vi "read shared memory.vi"(6 "channel classification":T1, 8 "error in":errorcluster, 10 "data table":T2, 11 "Shared Memory runtime":refnum<class "Shared Memory runtime.lvclass">) -> (0 "error out":errorcluster, 2 "data table out":T2, 3 "Shared Memory runtime out":refnum<class "Shared Memory runtime.lvclass">)   [LabVIEW 2014, in "Shared Memory runtime.lvclass"]
uses:
  Shared Memory runtime.lvclass
  <vilib>/NI/Tag Bus/table/data table.ctl
  <vilib>/NI/Tag Bus Module Framework/channel/channel classification.ctl
  Shared Memory runtime.lvclass/Shared Memory runtime.ctl
  <vilib>/NI/Tag Bus/table/data polymorphs/write many/write Doubles.vi
  <vilib>/NI/Tag Bus/table/data polymorphs/write many/write Singles.vi
  <vilib>/NI/Tag Bus/table/data polymorphs/write many/write I64s.vi
  <vilib>/NI/Tag Bus/table/data polymorphs/write many/write I32s.vi
  <vilib>/NI/Tag Bus/table/data polymorphs/write many/write I16s.vi
  <vilib>/NI/Tag Bus/table/data polymorphs/write many/write I8s.vi
  <vilib>/NI/Tag Bus/table/data polymorphs/write many/write U64s.vi
  <vilib>/NI/Tag Bus/table/data polymorphs/write many/write U32s.vi
  <vilib>/NI/Tag Bus/table/data polymorphs/write many/write U16s.vi
  <vilib>/NI/Tag Bus/table/data polymorphs/write many/write U8s.vi
  <vilib>/NI/Tag Bus/table/data polymorphs/write many/write Booleans.vi
  <vilib>/NI/Tag Bus/table/data polymorphs/write sequential/write sequential Doubles.vi
  <vilib>/NI/Tag Bus/table/data polymorphs/write sequential/write sequential Singles.vi
  <vilib>/NI/Tag Bus/table/data polymorphs/write sequential/write sequential I64s.vi
  <vilib>/NI/Tag Bus/table/data polymorphs/write sequential/write sequential I32s.vi
  <vilib>/NI/Tag Bus/table/data polymorphs/write sequential/write sequential I16s.vi
  <vilib>/NI/Tag Bus/table/data polymorphs/write sequential/write sequential I8s.vi
  <vilib>/NI/Tag Bus/table/data polymorphs/write sequential/write sequential U64s.vi
  <vilib>/NI/Tag Bus/table/data polymorphs/write sequential/write sequential U32s.vi
  <vilib>/NI/Tag Bus/table/data polymorphs/write sequential/write sequential U16s.vi
  <vilib>/NI/Tag Bus/table/data polymorphs/write sequential/write sequential U8s.vi
  <vilib>/NI/Tag Bus/table/data polymorphs/write sequential/write sequential Booleans.vi
  Read input data.vi
  Read processing parameters.vi
  Read processing results.vi
  Read output data.vi
  <vilib>/NI/NI Linux RT IPC/Shared Memory/Classes/Shared Memory/Shared Memory.lvclass
  <vilib>/NI/Tag Bus/table/data table.lvlib
  <vilib>/NI/NI Linux RT IPC/Shared Memory/Shared Memory.lvlib
  <vilib>/NI/Tag Bus Module Framework/channel/TBM channel.lvclass
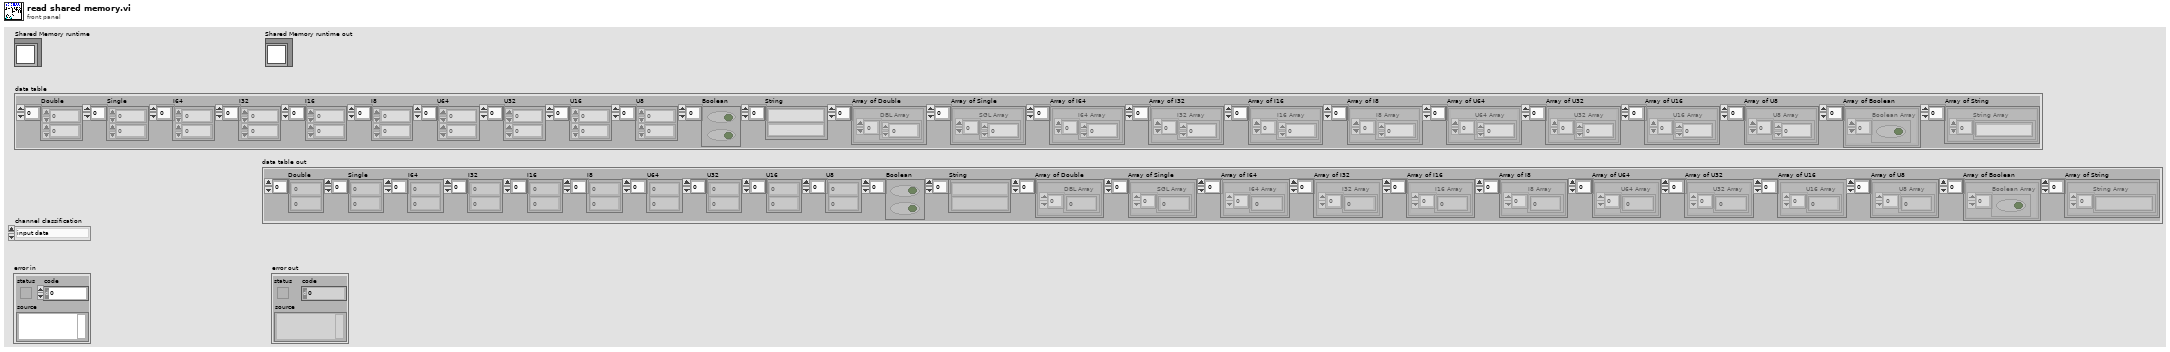
[diagram p1: front panel]
types:
  T1 = typedef "TBM channel.lvclass/channel classification.ctl" = enum16{"input data", "output data", "processing parameter", "processing result"}
  T2 = typedef "tag bus.lvlib/data table.lvlib/data table.ctl" = cluster{"Double":dbl[], "Single":sgl[], "I64":i64[], "I32":i32[], "I16":i16[], "I8":i8[], "U64":u64[], "U32":u32[], "U16":u16[], "U8":u8[], "Boolean":bool[], "String":string[], "Array of Double":cluster{"DBL Array":dbl[]}[], "Array of Single":cluster{"SGL Array":sgl[]}[], "Array of I64":cluster{"I64 Array":i64[]}[], "Array of I32":cluster{"I32 Array":i32[]}[], "Array of I16":cluster{"I16 Array":i16[]}[], "Array of I8":cluster{"I8 Array":i8[]}[], "Array of U64":cluster{"U64 Array":u64[]}[], "Array of U32":cluster{"U32 Array":u32[]}[], "Array of U16":cluster{"U16 Array":u16[]}[], "Array of U8":cluster{"U8 Array":u8[]}[], "Array of Boolean":cluster{"Boolean Array":bool[]}[], "Array of String":cluster{"String Array":string[]}[]}
  T3 = typedef "Shared Memory runtime.lvclass/channel runtime.ctl" = cluster{"channel classification":T1, "data type":T4, "pointer to shared memory":u64, "number of elements":u64, "data dictionary index":cluster{i32[]}, "shared memory":T5, "first tag index":i32, "sequential tags?":bool}
  T4 = typedef "tag bus.lvlib/tag descriptor.lvclass/Data Type.ctl" = enum16{"Double", "Single", "I64", "I32", "I16", "I8", "U64", "U32", "U16", "U8", "Boolean", "String", "Array of Double", "Array of Single", "Array of I64", "Array of I32", "Array of I16", "Array of I8", "Array of U64", "Array of U32", "Array of U16", "Array of U8", "Array of Boolean", "Array of String"}
  T5 = typedef "Linux RT IPC.lvlib/Shared Memory.lvlib/reference.ctl" = refnum<data-value>
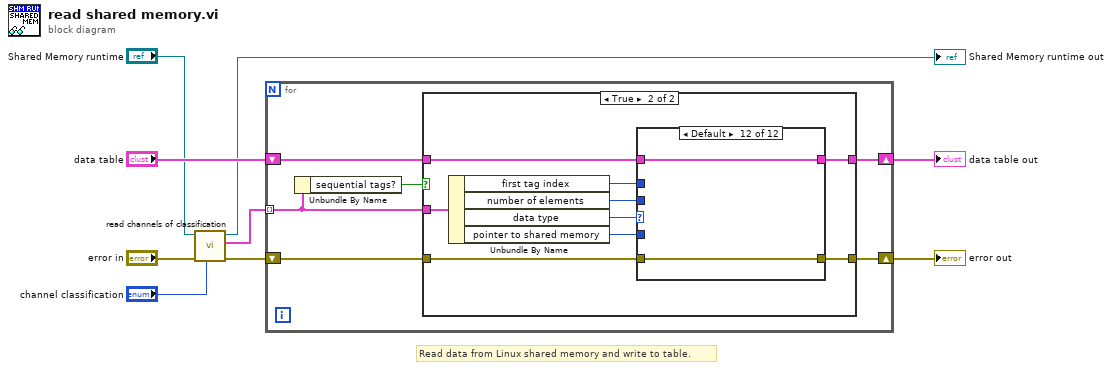
[diagram p0: block diagram]
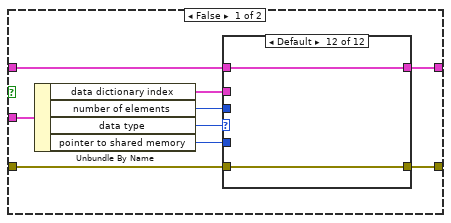
[diagram p2: hidden frame]
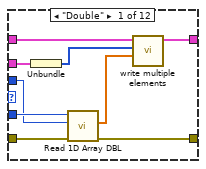
[diagram p3: hidden frame]
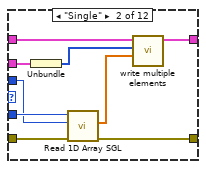
[diagram p4: hidden frame]
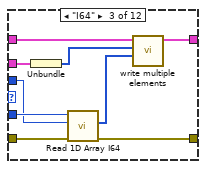
[diagram p5: hidden frame]
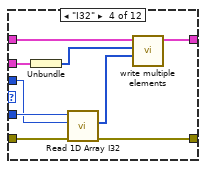
[diagram p6: hidden frame]
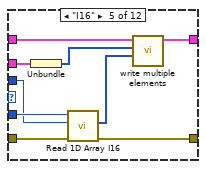
[diagram p7: hidden frame]
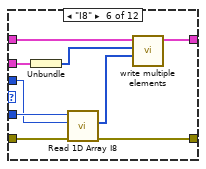
[diagram p8: hidden frame]
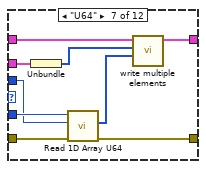
[diagram p9: hidden frame]
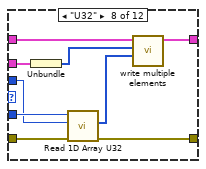
[diagram p10: hidden frame]
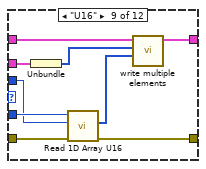
[diagram p11: hidden frame]
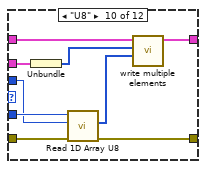
[diagram p12: hidden frame]
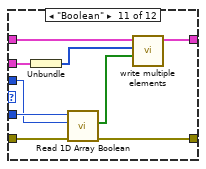
[diagram p13: hidden frame]
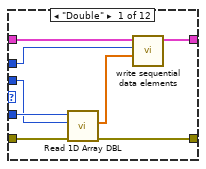
[diagram p14: hidden frame]
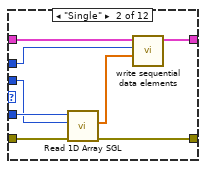
[diagram p15: hidden frame]
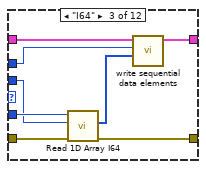
[diagram p16: hidden frame]
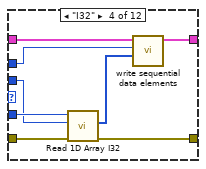
[diagram p17: hidden frame]
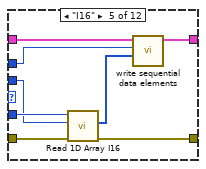
[diagram p18: hidden frame]
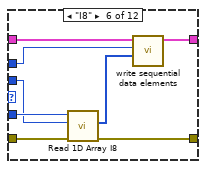
[diagram p19: hidden frame]
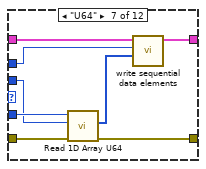
[diagram p20: hidden frame]
diagram:
  # "Read data from Linux shared memory and write to table."
  n1 = call "read channels of classification.vi"("channel classification"="channel classification", "error in"="error in", "Shared Memory runtime in"="Shared Memory runtime") -> ("error out"=w9:errorcluster, "channels"=w8:T3[], "Shared Memory runtime out"=→"Shared Memory runtime out":refnum<class "Shared Memory runtime.lvclass">)  [unwired: 6 in]
  n2 = for {
    tunnel: w8 -> [w11] mode=indexing
    shift-right: [w12] -> w5
    shift-left: w9 -> [w13]
    shift-right: [w15] -> w4
    shift-left: "data table" -> [w14]
    # "Write data from data table to Linux shared memory."
    n3 = Unbundle By Name(w11) -> ("sequential tags?"=w10:bool)
    n4 = case shown="True" w10 {
      tunnel: [w20 w130] -> w15
      tunnel: w14 -> [w21 w131]
      tunnel: w13 -> [w23 w133]
      tunnel: [w22 w132] -> w12
      tunnel: w11 -> [w24 w134]
      frame False {
        n5 = Unbundle By Name(w24) -> ("data dictionary index"=w17:cluster{i32[]}, "number of elements"=w16:u64, "data type"=w18:T4, "pointer to shared memory"=w19:u64)
        n6 = case shown="Default" w18 {
          tunnel: w21 -> [w33 w42 w51 w60 w69 w78 w87 w96 w105 w114 w123 w125]
          tunnel: [w32 w41 w50 w59 w68 w77 w86 w95 w104 w113 w122 w125] -> w20
          tunnel: w23 -> [w30 w39 w48 w57 w66 w75 w84 w93 w102 w111 w121 w124]
          tunnel: [w29 w38 w47 w56 w65 w74 w83 w92 w101 w110 w120 w124] -> w22
          tunnel: w19 -> [w28 w35 w44 w53 w63 w71 w80 w89 w98 w107 w118 _]
          tunnel: w17 -> [w26 w37 w46 w55 w64 w73 w82 w90 w100 w109 w116 _]
          tunnel: w16 -> [w27 w34 w43 w52 w62 w70 w79 w88 w97 w106 w117 _]
          frame "Double" {
            n7 = Unbundle(w26) -> (w25:i32[])
            n8 = call <vilib>:"Read 1D Array DBL.vi"("error in (no error)"=w30, "number of elements"=w27, "pointer in"=w28) -> ("error out"=w29:errorcluster, "value"=w31:dbl[])  [unwired: 6 in, 1 out]
            n9 = call-poly <vilib>:"write multiple elements.vi"("values"=w31, "indices"=w25, "data table in"=w33) -> ("data table out"=w32:T2)  [unwired: 8 in]
          }
          frame "Single" {
            n10 = Unbundle(w37) -> (w36:i32[])
            n11 = call <vilib>:"Read 1D Array SGL.vi"("error in (no error)"=w39, "number of elements"=w34, "pointer in"=w35) -> ("error out"=w38:errorcluster, "value"=w40:sgl[])  [unwired: 6 in, 1 out]
            n12 = call-poly <vilib>:"write multiple elements.vi"("values"=w40, "indices"=w36, "data table in"=w42) -> ("data table out"=w41:T2)  [unwired: 8 in]
          }
          frame "I64" {
            n13 = Unbundle(w46) -> (w45:i32[])
            n14 = call <vilib>:"Read 1D Array I64.vi"("error in (no error)"=w48, "number of elements"=w43, "pointer in"=w44) -> ("error out"=w47:errorcluster, "value"=w49:i64[])  [unwired: 6 in, 1 out]
            n15 = call-poly <vilib>:"write multiple elements.vi"("values"=w49, "indices"=w45, "data table in"=w51) -> ("data table out"=w50:T2)  [unwired: 8 in]
          }
          frame "I32" {
            n16 = Unbundle(w55) -> (w54:i32[])
            n17 = call <vilib>:"Read 1D Array I32.vi"("error in (no error)"=w57, "number of elements"=w52, "pointer in"=w53) -> ("error out"=w56:errorcluster, "value"=w58:i32[])  [unwired: 6 in, 1 out]
            n18 = call-poly <vilib>:"write multiple elements.vi"("values"=w58, "indices"=w54, "data table in"=w60) -> ("data table out"=w59:T2)  [unwired: 8 in]
          }
          frame "I16" {
            n19 = Unbundle(w64) -> (w61:i32[])
            n20 = call <vilib>:"Read 1D Array I16.vi"("error in (no error)"=w66, "number of elements"=w62, "pointer in"=w63) -> ("error out"=w65:errorcluster, "value"=w67:i16[])  [unwired: 6 in, 1 out]
            n21 = call-poly <vilib>:"write multiple elements.vi"("values"=w67, "indices"=w61, "data table in"=w69) -> ("data table out"=w68:T2)  [unwired: 8 in]
          }
          frame "I8" {
            n22 = Unbundle(w73) -> (w72:i32[])
            n23 = call <vilib>:"Read 1D Array I8.vi"("error in (no error)"=w75, "number of elements"=w70, "pointer in"=w71) -> ("error out"=w74:errorcluster, "value"=w76:i8[])  [unwired: 6 in, 1 out]
            n24 = call-poly <vilib>:"write multiple elements.vi"("values"=w76, "indices"=w72, "data table in"=w78) -> ("data table out"=w77:T2)  [unwired: 8 in]
          }
          frame "U64" {
            n25 = Unbundle(w82) -> (w81:i32[])
            n26 = call <vilib>:"Read 1D Array U64.vi"("error in (no error)"=w84, "number of elements"=w79, "pointer in"=w80) -> ("error out"=w83:errorcluster, "value"=w85:u64[])  [unwired: 6 in, 1 out]
            n27 = call-poly <vilib>:"write multiple elements.vi"("values"=w85, "indices"=w81, "data table in"=w87) -> ("data table out"=w86:T2)  [unwired: 8 in]
          }
          frame "U32" {
            n28 = Unbundle(w90) -> (w91:i32[])
            n29 = call <vilib>:"Read 1D Array U32.vi"("error in (no error)"=w93, "number of elements"=w88, "pointer in"=w89) -> ("error out"=w92:errorcluster, "value"=w94:u32[])  [unwired: 6 in, 1 out]
            n30 = call-poly <vilib>:"write multiple elements.vi"("values"=w94, "indices"=w91, "data table in"=w96) -> ("data table out"=w95:T2)  [unwired: 8 in]
          }
          frame "U16" {
            n31 = Unbundle(w100) -> (w99:i32[])
            n32 = call <vilib>:"Read 1D Array U16.vi"("error in (no error)"=w102, "number of elements"=w97, "pointer in"=w98) -> ("error out"=w101:errorcluster, "value"=w103:u16[])  [unwired: 6 in, 1 out]
            n33 = call-poly <vilib>:"write multiple elements.vi"("values"=w103, "indices"=w99, "data table in"=w105) -> ("data table out"=w104:T2)  [unwired: 8 in]
          }
          frame "U8" {
            n34 = Unbundle(w109) -> (w108:i32[])
            n35 = call <vilib>:"Read 1D Array U8.vi"("error in (no error)"=w111, "number of elements"=w106, "pointer in"=w107) -> ("error out"=w110:errorcluster, "value"=w112:u8[])  [unwired: 6 in, 1 out]
            n36 = call-poly <vilib>:"write multiple elements.vi"("values"=w112, "indices"=w108, "data table in"=w114) -> ("data table out"=w113:T2)  [unwired: 8 in]
          }
          frame "Boolean" {
            n37 = Unbundle(w116) -> (w115:i32[])
            n38 = call <vilib>:"Read 1D Array Boolean.vi"("error in (no error)"=w121, "number of elements"=w117, "pointer in"=w118) -> ("error out"=w120:errorcluster, "value"=w119:bool[])  [unwired: 6 in, 1 out]
            n39 = call-poly <vilib>:"write multiple elements.vi"("values"=w119, "indices"=w115, "data table in"=w123) -> ("data table out"=w122:T2)  [unwired: 8 in]
          }
          frame Default {
          }
        }
      }
      frame True {
        n40 = Unbundle By Name(w134) -> ("first tag index"=w127:i32, "number of elements"=w126:u64, "data type"=w128:T4, "pointer to shared memory"=w129:u64)
        n41 = case shown="Default" w128 {
          tunnel: w131 -> [w142 w150 w158 w166 w174 w182 w190 w198 w206 w214 w222 w224]
          tunnel: [w141 w149 w157 w165 w173 w181 w189 w197 w205 w213 w221 w224] -> w130
          tunnel: w133 -> [w139 w147 w155 w163 w171 w179 w187 w195 w203 w211 w220 w223]
          tunnel: [w138 w146 w154 w162 w170 w178 w186 w194 w202 w210 w219 w223] -> w132
          tunnel: w129 -> [w137 w145 w153 w161 w169 w177 w185 w193 w201 w209 w218 _]
          tunnel: w127 -> [w135 w143 w151 w159 w167 w175 w183 w191 w199 w207 w215 _]
          tunnel: w126 -> [w136 w144 w152 w160 w168 w176 w184 w192 w200 w208 w217 _]
          frame "Double" {
            n42 = call <vilib>:"Read 1D Array DBL.vi"("error in (no error)"=w139, "number of elements"=w136, "pointer in"=w137) -> ("error out"=w138:errorcluster, "value"=w140:dbl[])  [unwired: 6 in, 1 out]
            n43 = call-poly <vilib>:"write sequential data elements.vi"("values"=w140, "index"=w135, "data table in"=w142) -> ("data table out"=w141:T2)  [unwired: 8 in]
          }
          frame "Single" {
            n44 = call <vilib>:"Read 1D Array SGL.vi"("error in (no error)"=w147, "number of elements"=w144, "pointer in"=w145) -> ("error out"=w146:errorcluster, "value"=w148:sgl[])  [unwired: 6 in, 1 out]
            n45 = call-poly <vilib>:"write sequential data elements.vi"("values"=w148, "index"=w143, "data table in"=w150) -> ("data table out"=w149:T2)  [unwired: 8 in]
          }
          frame "I64" {
            n46 = call <vilib>:"Read 1D Array I64.vi"("error in (no error)"=w155, "number of elements"=w152, "pointer in"=w153) -> ("error out"=w154:errorcluster, "value"=w156:i64[])  [unwired: 6 in, 1 out]
            n47 = call-poly <vilib>:"write sequential data elements.vi"("values"=w156, "index"=w151, "data table in"=w158) -> ("data table out"=w157:T2)  [unwired: 8 in]
          }
          frame "I32" {
            n48 = call <vilib>:"Read 1D Array I32.vi"("error in (no error)"=w163, "number of elements"=w160, "pointer in"=w161) -> ("error out"=w162:errorcluster, "value"=w164:i32[])  [unwired: 6 in, 1 out]
            n49 = call-poly <vilib>:"write sequential data elements.vi"("values"=w164, "index"=w159, "data table in"=w166) -> ("data table out"=w165:T2)  [unwired: 8 in]
          }
          frame "I16" {
            n50 = call <vilib>:"Read 1D Array I16.vi"("error in (no error)"=w171, "number of elements"=w168, "pointer in"=w169) -> ("error out"=w170:errorcluster, "value"=w172:i16[])  [unwired: 6 in, 1 out]
            n51 = call-poly <vilib>:"write sequential data elements.vi"("values"=w172, "index"=w167, "data table in"=w174) -> ("data table out"=w173:T2)  [unwired: 8 in]
          }
          frame "I8" {
            n52 = call <vilib>:"Read 1D Array I8.vi"("error in (no error)"=w179, "number of elements"=w176, "pointer in"=w177) -> ("error out"=w178:errorcluster, "value"=w180:i8[])  [unwired: 6 in, 1 out]
            n53 = call-poly <vilib>:"write sequential data elements.vi"("values"=w180, "index"=w175, "data table in"=w182) -> ("data table out"=w181:T2)  [unwired: 8 in]
          }
          frame "U64" {
            n54 = call <vilib>:"Read 1D Array U64.vi"("error in (no error)"=w187, "number of elements"=w184, "pointer in"=w185) -> ("error out"=w186:errorcluster, "value"=w188:u64[])  [unwired: 6 in, 1 out]
            n55 = call-poly <vilib>:"write sequential data elements.vi"("values"=w188, "index"=w183, "data table in"=w190) -> ("data table out"=w189:T2)  [unwired: 8 in]
          }
          frame "U32" {
            n56 = call <vilib>:"Read 1D Array U32.vi"("error in (no error)"=w195, "number of elements"=w192, "pointer in"=w193) -> ("error out"=w194:errorcluster, "value"=w196:u32[])  [unwired: 6 in, 1 out]
            n57 = call-poly <vilib>:"write sequential data elements.vi"("values"=w196, "index"=w191, "data table in"=w198) -> ("data table out"=w197:T2)  [unwired: 8 in]
          }
          frame "U16" {
            n58 = call <vilib>:"Read 1D Array U16.vi"("error in (no error)"=w203, "number of elements"=w200, "pointer in"=w201) -> ("error out"=w202:errorcluster, "value"=w204:u16[])  [unwired: 6 in, 1 out]
            n59 = call-poly <vilib>:"write sequential data elements.vi"("values"=w204, "index"=w199, "data table in"=w206) -> ("data table out"=w205:T2)  [unwired: 8 in]
          }
          frame "U8" {
            n60 = call <vilib>:"Read 1D Array U8.vi"("error in (no error)"=w211, "number of elements"=w208, "pointer in"=w209) -> ("error out"=w210:errorcluster, "value"=w212:u8[])  [unwired: 6 in, 1 out]
            n61 = call-poly <vilib>:"write sequential data elements.vi"("values"=w212, "index"=w207, "data table in"=w214) -> ("data table out"=w213:T2)  [unwired: 8 in]
          }
          frame "Boolean" {
            n62 = call <vilib>:"Read 1D Array Boolean.vi"("error in (no error)"=w220, "number of elements"=w217, "pointer in"=w218) -> ("error out"=w219:errorcluster, "value"=w216:bool[])  [unwired: 6 in, 1 out]
            n63 = call-poly <vilib>:"write sequential data elements.vi"("values"=w216, "index"=w215, "data table in"=w222) -> ("data table out"=w221:T2)  [unwired: 8 in]
          }
          frame Default {
          }
        }
      }
    }
  }
  "error out" <- w5
  "data table out" <- w4
